vi "XY Graph Get Caption (or Label).vi"(8 "error in (no error)":errorcluster, 11 "XYGraph in":T1) -> (0 "error out":errorcluster, 2 "Caption (or Label) Text":string, 3 "XYGraph out":T1)   [LabVIEW 2019, in "XY Graph Add-Ons.lvlib"]
uses:
  XY Graph Add-Ons.lvlib
  XY Graph Refnum.ctl
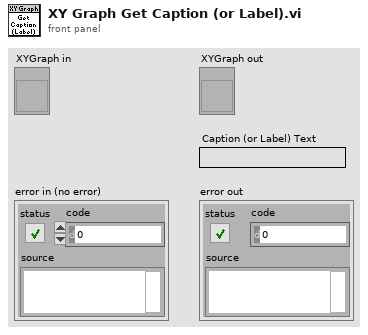
[diagram p1: front panel]
types:
  T1 = typedef "XY Graph Add-Ons.lvlib/XY Graph Refnum.ctl" = refnum<vi>
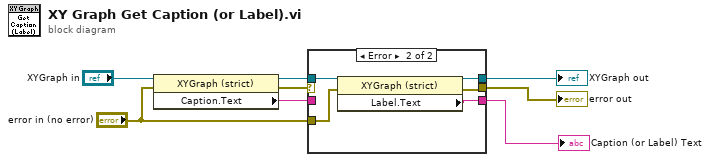
[diagram p0: block diagram]
diagram:
  n1 = property class="XYGraph (strict)"(reference="XYGraph in", error in="error in (no error)") -> (reference out=w5:T1, error out=w2:errorcluster, "Caption.Text"=w3:string)
  n2 = case shown="Error" w2 {
    selector: w2 -> [w10 _]
    tunnel: w3 -> [w11 _]
    tunnel: [w11 w12] -> w4
    tunnel: w5 -> [w9 w16]
    tunnel: [w10 w13] -> w8
    tunnel: [w9 w14] -> w6
    tunnel: "error in (no error)" -> [_ w15]
    frame No Error {
    }
    frame Error {
      n3 = property class="XYGraph (strict)"(reference=w16, error in=w15) -> (reference out=w14:T1, error out=w13:errorcluster, "Label.Text"=w12:string)
    }
  }
  "error out" <- w8
  "XYGraph out" <- w6
  "Caption (or Label) Text" <- w4
